vi "DrawMenuItems.vi"(8 "error in (no error)":errorcluster, 11 "menu in":refnum<class "menu.lvclass">) -> (0 "error out":errorcluster, 3 "menu out":refnum<class "menu.lvclass">)   [LabVIEW 2009, in "menu.lvclass"]
uses:
  menu.lvclass
  menu.lvclass/menu.ctl
  Menu Item/menu item.lvclass
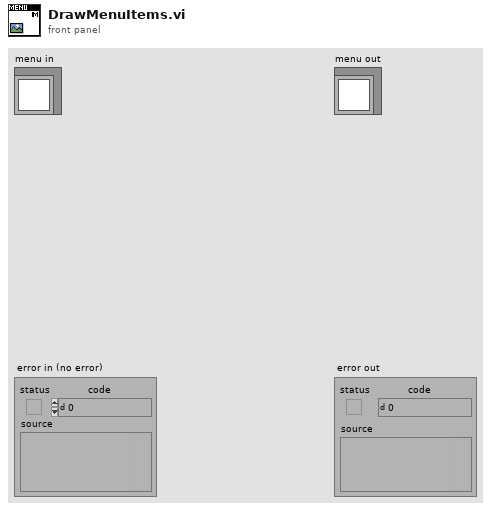
[diagram p1: front panel]
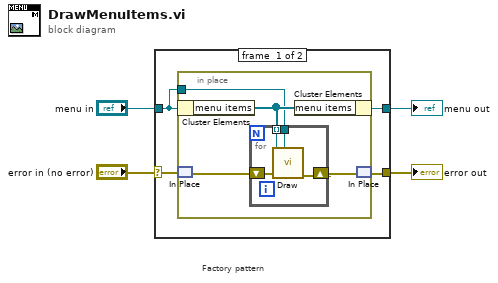
[diagram p0: block diagram]
diagram:
  # "Factory pattern"
  n1 = case shown="No Error" "error in (no error)" {
    selector: "error in (no error)" -> [w7 w18]
    tunnel: [w6 w18] -> w1
    tunnel: [w8 w17] -> w3
    tunnel: "menu in" -> [w5 w17]
    frame #0 {
      n2 = in-place {
        in-place-border: w5 -> [w11]
        n3 = in-place-cluster #1(w5) -> ("menu items"=w12:refnum<class "menu item.lvclass">[])
        n4 = in-place-match #2(w7) -> (w10:errorcluster)
        n5 = for {
          tunnel: w11 -> [w16]
          tunnel: w12 -> [w15] mode=indexing
          shift-right: [w13] -> w9
          shift-left: w10 -> [w14]
          n6 = call-dynamic "Draw.vi"("menu in"=w16, "error in (no error)"=w14, "menu item in"=w15) -> ("error out"=w13:errorcluster)  [unwired: 7 in, 1 out]
        }
        n7 = in-place-cluster #1("menu items"=w12) -> (w8:refnum<class "menu.lvclass">)
        n8 = in-place-match #2(w9) -> (w6:errorcluster)
      }
    }
    frame #1 {
    }
  }
  "menu out" <- w3
  "error out" <- w1
